vi "clearEvents.vi"(8 "error in (no error)":errorcluster, 11 "SM1000-control in":T1) -> (0 "error out":errorcluster, 3 "SM1000-control out":T1)   [LabVIEW 2013, in "SLMControl.lvlib" / "SM1000.lvclass"]
doc: "Unregisters the application for 'OnConnect'-events."
uses:
  SM1000.lvclass
  Object-reference.ctl
  SM1000.lvclass/SM1000.ctl
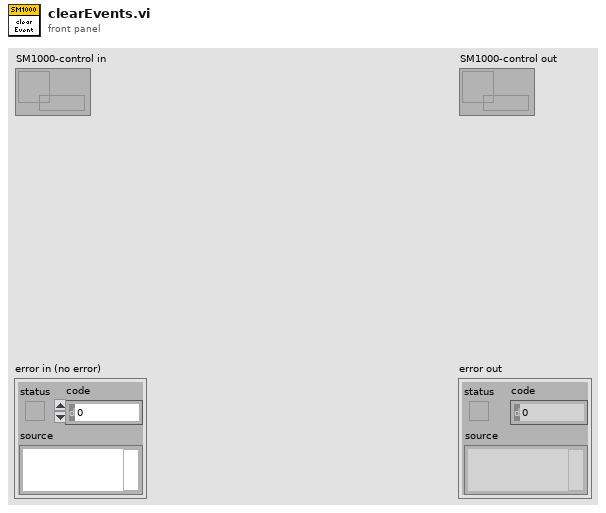
[diagram p1: front panel]
types:
  T1 = typedef "SLMControl.lvlib/SM1000.lvclass/Object-reference.ctl" = refnum<data-value>
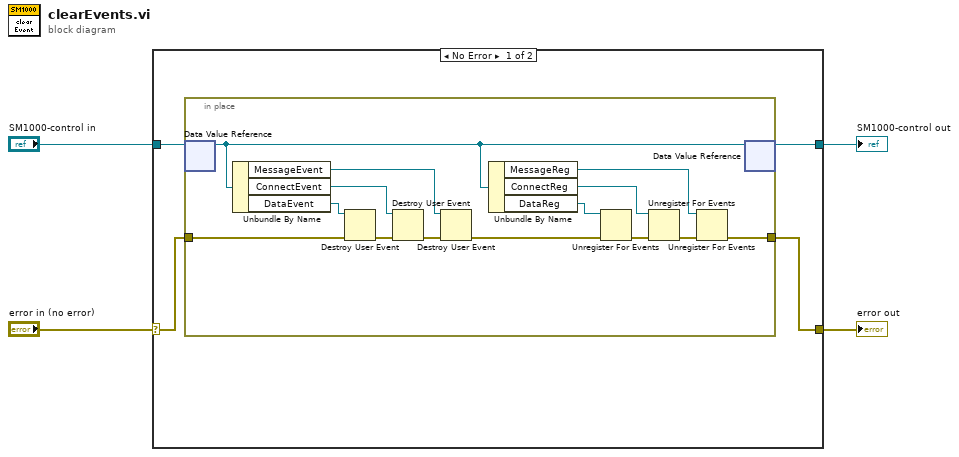
[diagram p0: block diagram]
diagram:
  n1 = case shown="No Error" "error in (no error)" {
    selector: "error in (no error)" -> [w5 w24]
    tunnel: [w6 w24] -> w3
    tunnel: [w7 w23] -> w1
    tunnel: "SM1000-control in" -> [w8 w23]
    frame No Error {
      n2 = in-place {
        in-place-border: w5 -> [w17]
        in-place-border: [w12] -> w6
        n3 = in-place-dvr #1(w8) -> (w16:refnum<class "SM1000.lvclass">)  [unwired: 1 out]
        n4 = Unbundle By Name(w16) -> ("MessageEvent"=w18:refnum<user-event>, "ConnectEvent"=w20:refnum<user-event>, "DataEvent"=w22:refnum<user-event>)
        n5 = Destroy User Event(user event=w22, error in=w17) -> (error out=w21:errorcluster)
        n6 = Destroy User Event(user event=w20, error in=w21) -> (error out=w19:errorcluster)
        n7 = Destroy User Event(user event=w18, error in=w19) -> (error out=w15:errorcluster)
        n8 = Unbundle By Name(w16) -> ("MessageReg"=w9:refnum<k27>, "ConnectReg"=w10:refnum<k27>, "DataReg"=w11:refnum<k27>)
        n9 = Unregister For Events(event registration refnum=w11, error in=w15) -> (error out=w14:errorcluster)
        n10 = Unregister For Events(event registration refnum=w10, error in=w14) -> (error out=w13:errorcluster)
        n11 = Unregister For Events(event registration refnum=w9, error in=w13) -> (error out=w12:errorcluster)
        n12 = in-place-dvr #1(w16) -> (w7:T1)  [unwired: 1 out]
      }
    }
    frame Error {
    }
  }
  "error out" <- w3
  "SM1000-control out" <- w1
